vi "get image frame.vi"(0 "index":i32, 1 "fmt":T1(ring), 5 "error in (no error)":errorcluster) -> (10 "RGB Array":cluster{"R":u8, "G":u8, "B":u8}[](array[cluster]), 12 "YUB RGB Array":cluster{"R":u8, "G":u8, "B":u8}[](array[cluster]), 14 "Bayer Array":u8[](array[numeric]), 15 "IR 8Bit Array":u8[](array[numeric]), 16 "IR 10Bit Array":u16[](array[numeric]), 17 "YUB RAW Array":u16[](array[numeric]), 18 "IR 10Bit Packed Array":u8[](array[numeric]), 19 "error out":errorcluster)   [LabVIEW 2017, in "libfreenect.lvlib"]
doc: "EXPORT char *freenect_lv_get_image_frame(int index, freenect_video_format fmt);"
uses:
  libfreenect.lvlib
  freenect_lv.dll
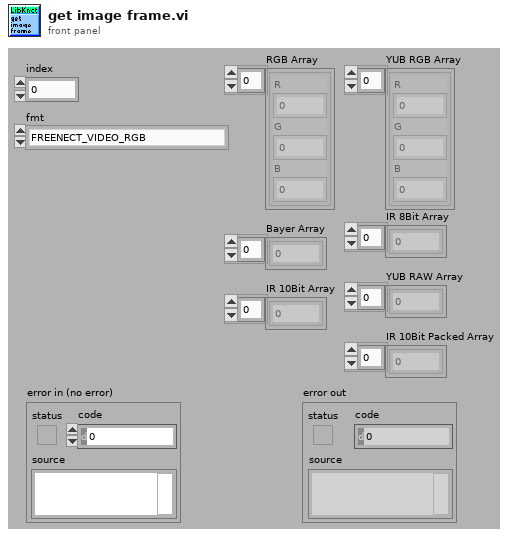
[diagram p1: front panel]
types:
  T1 = enum16{"FREENECT_VIDEO_RGB", "FREENECT_VIDEO_BAYER", "FREENECT_VIDEO_IR_8BIT", "FREENECT_VIDEO_IR_10BIT", "FREENECT_VIDEO_IR_10BIT_PACKED", "FREENECT_VIDEO_YUB_RGB", "FREENECT_VIDEO_YUB_RAW"}
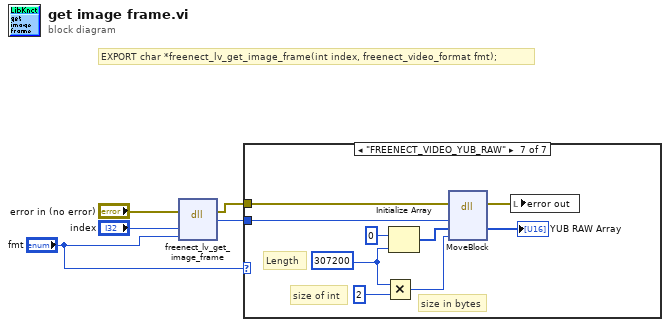
[diagram p0: block diagram]
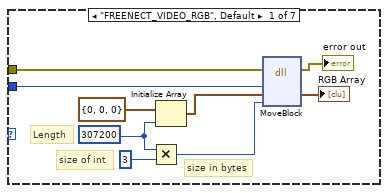
[diagram p2: hidden frame]
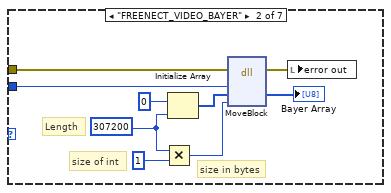
[diagram p3: hidden frame]
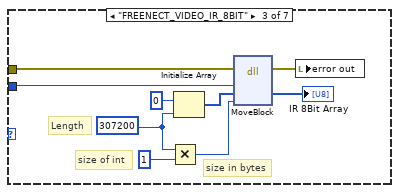
[diagram p4: hidden frame]
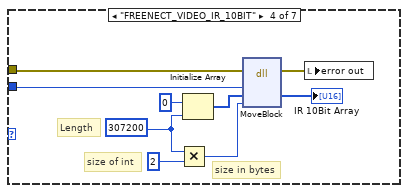
[diagram p5: hidden frame]
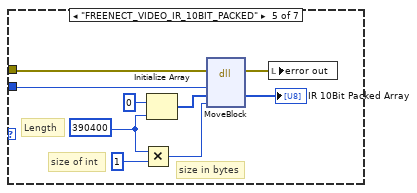
[diagram p6: hidden frame]
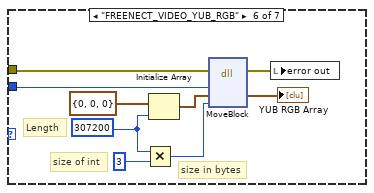
[diagram p7: hidden frame]
diagram:
  # "EXPORT char *freenect_lv_get_image_frame(int index, freenect_video_format fmt);"
  n1 = dll-call lib="C:/Users/Mats/Desktop/Bacheler prosjekt/Labview/Occupancy Grid Map Code - With model/freenect_lv.*" fn="freenect_lv_get_image_frame"(error in="error in (no error)", "index"="index", "fmt"="fmt") -> (error out=w1:errorcluster, "return type"=w2:i64)  [unwired: 3 in, 2 out]
  n2 = case shown="\"FREENECT_VIDEO_YUB_RAW\"" "fmt" {
    tunnel: w2 -> [w7 w19 w25 w33 w42 w53 w60]
    tunnel: w1 -> [w6 w20 w24 w34 w43 w54 w61]
    frame "FREENECT_VIDEO_RGB", Default {
      w12 = 307200 ("dimension size")
      # "size in bytes"
      # "size of int"
      # "Length"
      n3 = Multiply(x=w12, y=3) -> (x*y=w9:i32)
      n4 = Initialize Array(cluster{"R":u8, "G":u8, "B":u8} {"R"=0, "G"=0, "B"=0} ("RGB24bit"), w12) -> (w8:cluster{"R":u8, "G":u8, "B":u8}[])
      n5 = dll-call lib="LabVIEW" fn="MoveBlock"(error in=w6, "Address (Pointer)"=w7, "Destination"=w8, "Size"=w9) -> (error out=→"error out":errorcluster, "Destination"=→"RGB Array":cluster{"R":u8, "G":u8, "B":u8}[])  [unwired: 4 in, 2 out]
    }
    frame "FREENECT_VIDEO_BAYER" {
      w23 = 307200 ("dimension size")
      # "size in bytes"
      # "size of int"
      # "Length"
      n6 = Multiply(x=w23, y=1) -> (x*y=w21:i32)
      n7 = Initialize Array(u8 0, w23) -> (w18:u8[])
      n8 = dll-call lib="LabVIEW" fn="MoveBlock"(error in=w20, "Address (Pointer)"=w19, "Destination"=w18, "Size"=w21) -> (error out=w17:errorcluster, "Destination"=→"Bayer Array":u8[])  [unwired: 4 in, 2 out]
      n9 = local write "error out"(w17) -> ()
    }
    frame "FREENECT_VIDEO_IR_8BIT" {
      w28 = 307200 ("dimension size")
      # "size in bytes"
      # "size of int"
      # "Length"
      n10 = Multiply(x=w28, y=1) -> (x*y=w30:i32)
      n11 = Initialize Array(u8 0, w28) -> (w31:u8[])
      n12 = dll-call lib="LabVIEW" fn="MoveBlock"(error in=w24, "Address (Pointer)"=w25, "Destination"=w31, "Size"=w30) -> (error out=w32:errorcluster, "Destination"=→"IR 8Bit Array":u8[])  [unwired: 4 in, 2 out]
      n13 = local write "error out"(w32) -> ()
    }
    frame "FREENECT_VIDEO_IR_10BIT" {
      w39 = 307200 ("dimension size")
      # "size in bytes"
      # "size of int"
      # "Length"
      n14 = Multiply(x=w39, y=2) -> (x*y=w37:i32)
      n15 = Initialize Array(u16 0, w39) -> (w36:u16[])
      n16 = dll-call lib="LabVIEW" fn="MoveBlock"(error in=w34, "Address (Pointer)"=w33, "Destination"=w36, "Size"=w37) -> (error out=w35:errorcluster, "Destination"=→"IR 10Bit Array":u16[])  [unwired: 4 in, 2 out]
      n17 = local write "error out"(w35) -> ()
    }
    frame "FREENECT_VIDEO_IR_10BIT_PACKED" {
      w46 = 390400 ("dimension size")
      # "size in bytes"
      # "size of int"
      # "Length"
      n18 = Multiply(x=w46, y=1) -> (x*y=w48:i32)
      n19 = Initialize Array(u8 0, w46) -> (w49:u8[])
      n20 = dll-call lib="LabVIEW" fn="MoveBlock"(error in=w43, "Address (Pointer)"=w42, "Destination"=w49, "Size"=w48) -> (error out=w50:errorcluster, "Destination"=→"IR 10Bit Packed Array":u8[])  [unwired: 4 in, 2 out]
      n21 = local write "error out"(w50) -> ()
    }
    frame "FREENECT_VIDEO_YUB_RGB" {
      w59 = 307200 ("dimension size")
      # "size in bytes"
      # "size of int"
      # "Length"
      n22 = Multiply(x=w59, y=3) -> (x*y=w57:i32)
      n23 = Initialize Array(cluster{"R":u8, "G":u8, "B":u8} {"R"=0, "G"=0, "B"=0} ("RGB24bit"), w59) -> (w56:cluster{"R":u8, "G":u8, "B":u8}[])
      n24 = dll-call lib="LabVIEW" fn="MoveBlock"(error in=w54, "Address (Pointer)"=w53, "Destination"=w56, "Size"=w57) -> (error out=w55:errorcluster, "Destination"=→"YUB RGB Array":cluster{"R":u8, "G":u8, "B":u8}[])  [unwired: 4 in, 2 out]
      n25 = local write "error out"(w55) -> ()
    }
    frame "FREENECT_VIDEO_YUB_RAW" {
      w64 = 307200 ("dimension size")
      # "size in bytes"
      # "size of int"
      # "Length"
      n26 = Multiply(x=w64, y=2) -> (x*y=w66:i32)
      n27 = Initialize Array(u16 0, w64) -> (w67:u16[])
      n28 = dll-call lib="LabVIEW" fn="MoveBlock"(error in=w61, "Address (Pointer)"=w60, "Destination"=w67, "Size"=w66) -> (error out=w68:errorcluster, "Destination"=→"YUB RAW Array":u16[])  [unwired: 4 in, 2 out]
      n29 = local write "error out"(w68) -> ()
    }
  }
